vi "Load Framework.vi"(8 "error in (no error)":errorcluster, 11 "Application Refs":T1) -> (0 "error out":errorcluster, 3 "Application Data out":T1)   [LabVIEW 2017, in "DSF Core.lvlib"]
uses:
  DSF Core.lvlib
  Application Data.ctl
  <vilib>/NI/Memory Manager/Classes/Pointer/Pointer.lvclass
  Classes/Framework/Framework.lvclass
  Buffer Reader/Buffer Data.ctl
  Classes/Buffer/Buffer.lvclass
  Classes/Transfer Group Status/Status.lvclass
  Typedefs/DSF Engine Framework Configuration.ctl
  Typedefs/DSF Engine Plugin Configuration.ctl
  Typedefs/DSF Timing Info.ctl
  Typedefs/DSF Engine Plugin Thread Configuration.ctl
  Typedefs/DSF Settings Info.ctl
  Typedefs/DSF Engine Transfer Group Configuration.ctl
  Typedefs/DSF Direction.ctl
  Typedefs/DSF Engine Transfer Configuration.ctl
  Typedefs/DSF Byte Order.ctl
  Typedefs/DSF Engine Channel Configuration.ctl
  Typedefs/DSF Data Type.ctl
  Typedefs/DSF Timeout Behavior.ctl
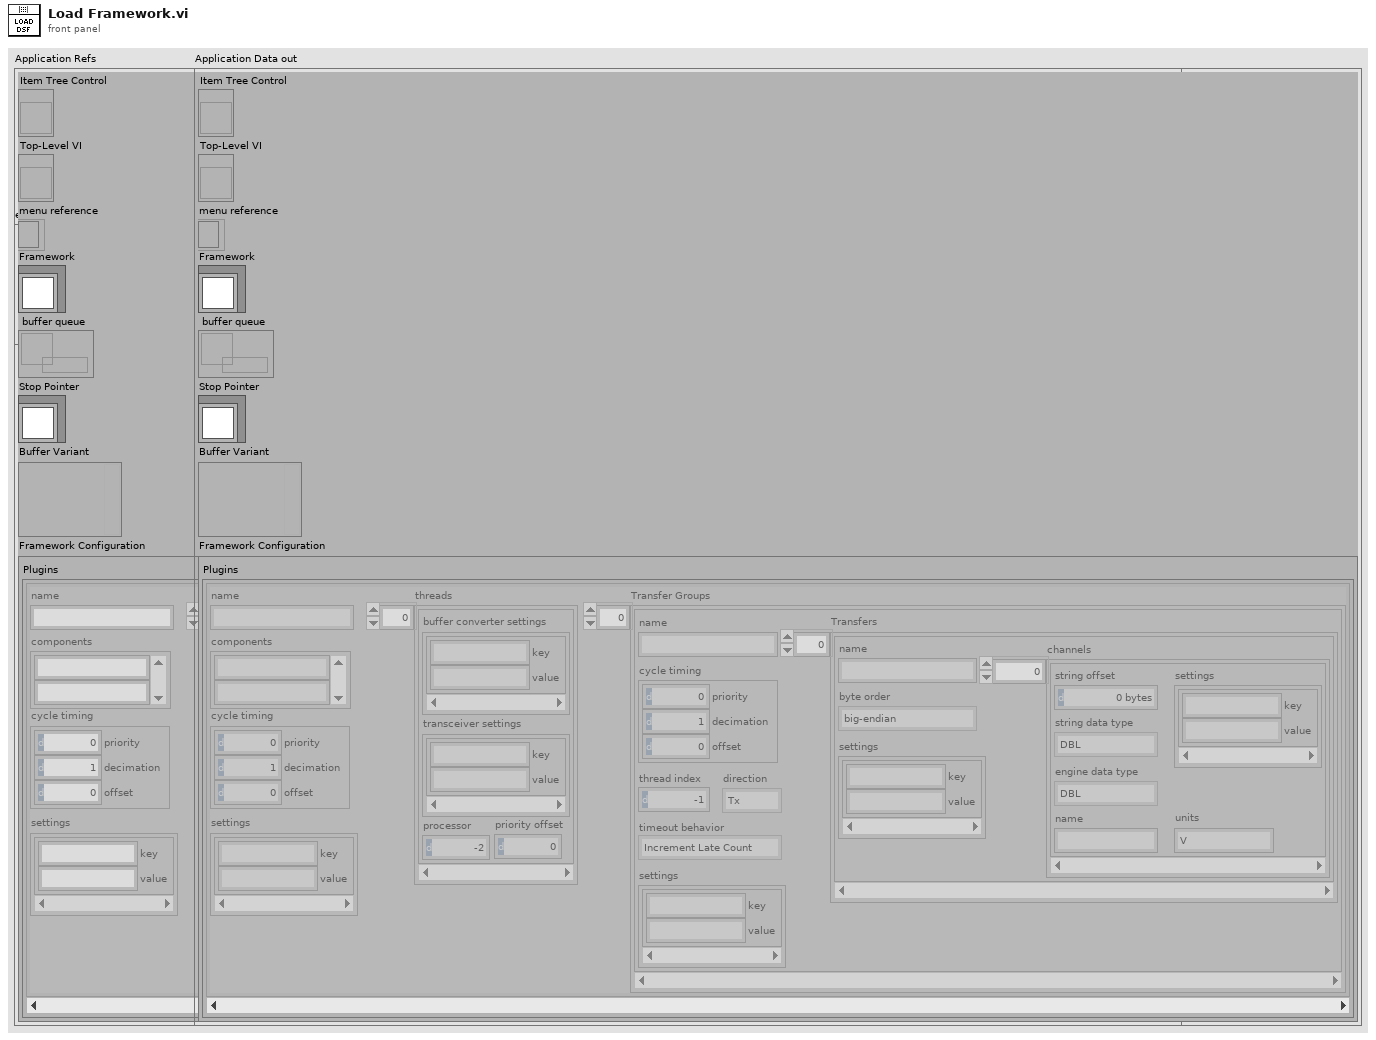
[diagram p1: front panel]
types:
  T1 = typedef "DSF Core.lvlib/Application Data.ctl" = cluster{"Item Tree Control":refnum<vi>, "Top-Level VI":refnum<vi>, "menu reference":refnum<k9>, "Framework":refnum<class "Framework.lvclass">, "buffer queue":refnum<queue>, "Stop Pointer":refnum<class "Pointer.lvclass">, "Buffer Variant":variant, "Framework Configuration":T2}
  T2 = typedef "DSF Core.lvlib/DSF Engine Framework Configuration.ctl" = cluster{"Plugins":T3[]}
  T3 = typedef "DSF Core.lvlib/DSF Engine Plugin Configuration.ctl" = cluster{"name":string, "components":string[], "cycle timing":T4, "threads":T5[], "Transfer Groups":T7[], "settings":T6}
  T4 = typedef "DSF Core.lvlib/DSF Timing Info.ctl" = cluster{"priority":u64, "decimation":u64, "offset":u64}
  T5 = typedef "DSF Core.lvlib/DSF Engine Plugin Thread Configuration.ctl" = cluster{"buffer converter settings":T6, "transceiver settings":T6, "processor":i32, "priority offset":i16}
  T6 = typedef "DSF Core.lvlib/DSF Settings Info.ctl" = cluster{"key":string, "value":string}[]
  T7 = typedef "DSF Core.lvlib/DSF Engine Transfer Group Configuration.ctl" = cluster{"name":string, "direction":T8, "cycle timing":T4, "thread index":i32, "settings":T6, "Transfers":T9[], "timeout behavior":T13}
  T8 = typedef "DSF Core.lvlib/DSF Direction.ctl" = enum8{"Tx", "Rx"}
  T9 = typedef "DSF Core.lvlib/DSF Engine Transfer Configuration.ctl" = cluster{"name":string, "byte order":T10, "settings":T6, "channels":T11[]}
  T10 = typedef "DSF Core.lvlib/DSF Byte Order.ctl" = enum8{"big-endian", "little-endian"}
  T11 = typedef "DSF Core.lvlib/DSF Engine Channel Configuration.ctl" = cluster{"string offset":u64, "string data type":T12, "engine data type":T12, "name":string, "settings":T6, "units":string}
  T12 = typedef "DSF Core.lvlib/DSF Data Type.ctl" = enum8{"Bool", "SGL", "DBL", "I8", "I16", "I32", "I64", "U8", "U16", "U32", "U64"}
  T13 = typedef "DSF Core.lvlib/DSF Timeout Behavior.ctl" = enum8{"Increment Late Count", "Throw Error"}
  T14 = typedef "DSF Core.lvlib/Buffer Data.ctl" = cluster{"Buffer":refnum<class "Buffer.lvclass">, "Status":refnum<class "Status.lvclass">, "decimation":u64, "avg bandwidth":dbl}
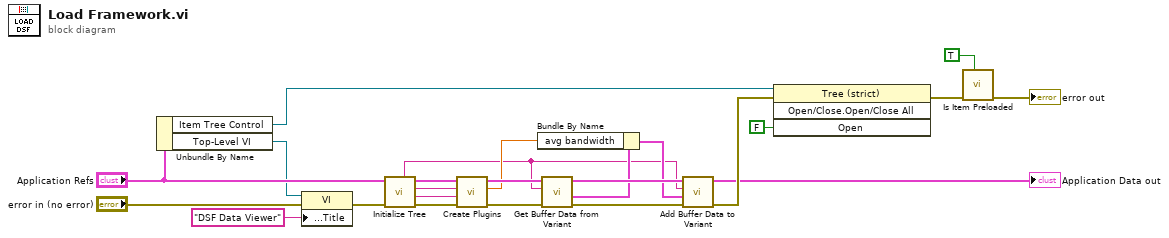
[diagram p0: block diagram]
diagram:
  n1 = Unbundle By Name("Application Refs") -> ("Item Tree Control"=w14:refnum<vi>, "Top-Level VI"=w1:refnum<vi>)
  n2 = property class="VI"(reference=w1, error in="error in (no error)", "Front Panel.Title"="DSF Data Viewer" ("Front Panel Window:Title")) -> (error out=w24:errorcluster)  [unwired: 1 out]
  n3 = call "Initialize Tree.vi"("error in (no error)"=w24, "Application Data in"="Application Refs") -> ("error out"=w17:errorcluster, "async plugins tag"=w15:string, "inline plugins tag"=w16:string, "Application Data out"=w18:T1, "framework tag"=w2:string)  [unwired: 5 in]
  n4 = call "Create Plugins.vi"("error in (no error)"=w17, "async plugins tag"=w15, "inline plugins tag"=w16, "Application Data In"=w18) -> ("error out"=w9:errorcluster, "avg bandwidth"=w4:dbl, "Application Data out"=w8:T1)  [unwired: 5 in]
  n5 = call "Get Buffer Data from Variant.vi"("error in (no error)"=w9, "tag"=w2, "Application Data In in"=w8) -> ("error out"=w6:errorcluster, "Buffer data"=w5:T14, "Application Data In out"=w7:T1)  [unwired: 6 in]
  n6 = Bundle By Name(cluster=w5, "avg bandwidth"=w4) -> (w3:T14)
  n7 = call "Add Buffer Data to Variant.vi"("error in (no error)"=w6, "Buffer data"=w3, "tag"=w2, "Application Data In in"=w7) -> ("error out"=w12:errorcluster, "Application Data In out"=→"Application Data out":T1)  [unwired: 6 in]
  n8 = invoke class="Tree (strict)" method="Open/Close.Open/Close All"(reference=w14, error in=w12, "Open"=FALSE ("Open?")) -> (error out=w11:errorcluster)  [unwired: 1 in, 3 out]
  n9 = call "Is Item Preloaded"("clear entries"=TRUE, "error in (no error)"=w11) -> ("error out"=→"error out":errorcluster)  [unwired: 7 in, 2 out]
